vi "Get Digital Pattern - Multi FPGA.vi"(8 "error in (no error)":errorcluster, 11 "Item Ref in":T1 format="%.0x") -> (0 "error out":errorcluster, 2 "EPT Pattern":T2, 3 "Item Ref out":T1 format="%.0x")   [LabVIEW 2019, in "Engine Simulation Toolkit System Explorer.lvlib"]
uses:
  Engine Simulation Toolkit System Explorer.lvlib
  <vilib>/NI VeriStand/Custom Device API/Custom Device Item Ref.ctl
  Digital Pattern.ctl
  Digital Pattern Base.ctl
  Digital Pattern Remove Edge.ctl
  Digital Pattern Add Pulse.ctl
  Shared/Properties.vi
  <vilib>/NI VeriStand/Custom Device API/Get Item Property (Double).vi
  <vilib>/NI VeriStand/Custom Device API/Get Item Property (U16).vi
  <vilib>/NI VeriStand/Custom Device API/Get Item Property (String).vi
  <vilib>/NI VeriStand/Custom Device API/Get Item Property (Boolean).vi
  <vilib>/NI VeriStand/Custom Device API/Custom Device API.lvlib
  Shared/Engine Simulation Toolkit Shared.lvlib
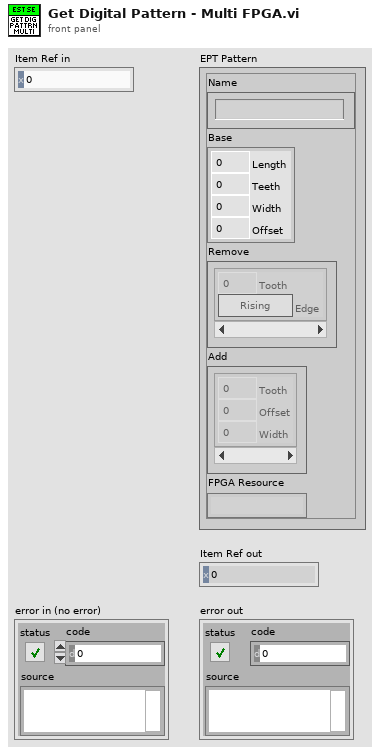
[diagram p1: front panel]
types:
  T1 = typedef "Custom Device API.lvlib/Custom Device Item Ref.ctl" = u64
  T2 = typedef "Engine Simulation Toolkit System Explorer.lvlib/Digital Pattern.ctl" = cluster{"Name":string, "Base":T3, "Remove":T4[], "Add":T5[], "FPGA Resource":string}
  T3 = typedef "Engine Simulation Toolkit System Explorer.lvlib/Digital Pattern Base.ctl" = cluster{"Length":dbl, "Teeth":u16, "Width":dbl, "Offset":dbl}
  T4 = typedef "Engine Simulation Toolkit System Explorer.lvlib/Digital Pattern Remove Edge.ctl" = cluster{"Tooth":u16, "Edge":bool}
  T5 = typedef "Engine Simulation Toolkit System Explorer.lvlib/Digital Pattern Add Pulse.ctl" = cluster{"Tooth":u16, "Offset":dbl, "Width":dbl}
  T6 = typedef "Custom Device API.lvlib/Custom Device Item Info.ctl" = cluster{"Name":string, "Is Channel":bool, "GUID":string, "Is Waveform":bool}
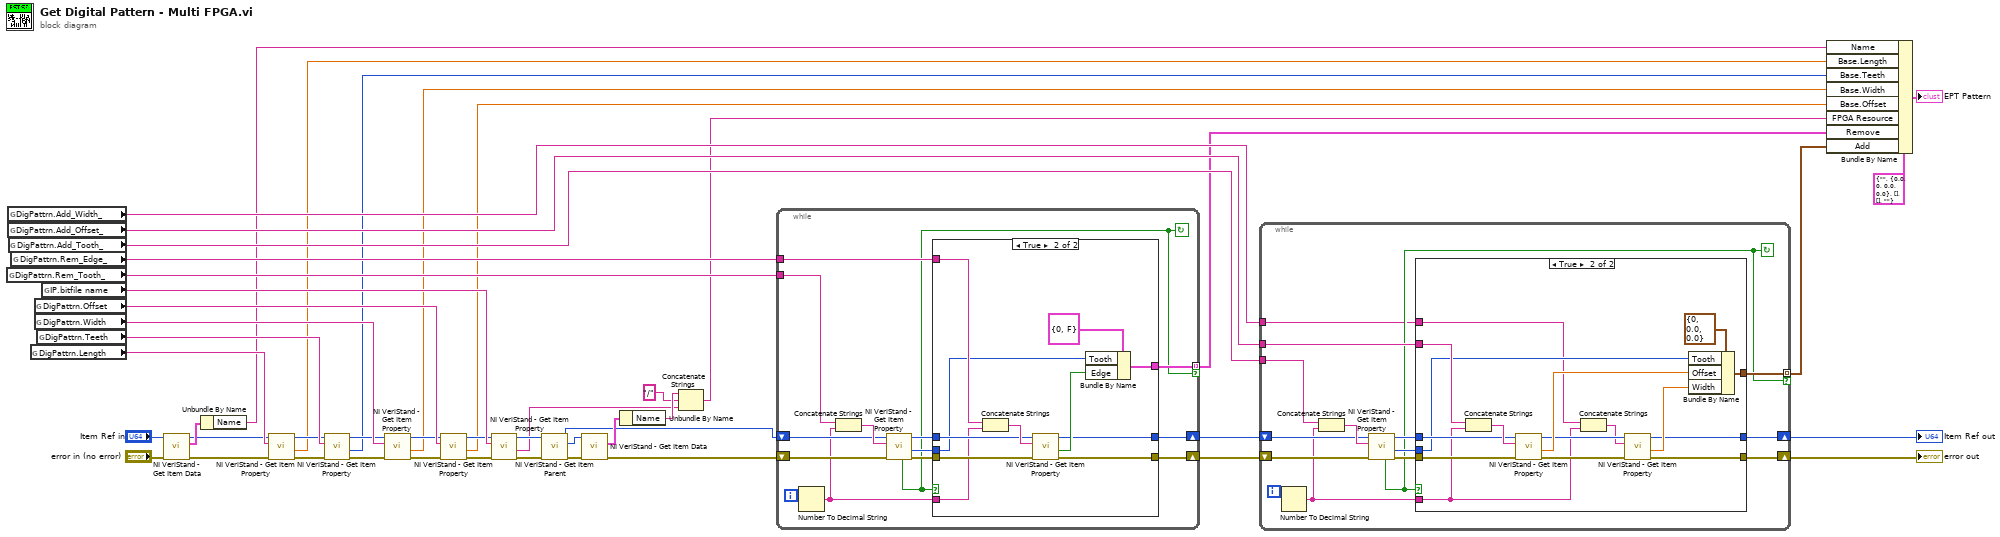
[diagram p0: block diagram]
diagram:
  n1 = global read "Properties.vi" "DigPattrn.Rem_Tooth_"() -> (w43:string)
  n2 = global read "Properties.vi" "DigPattrn.Add_Width_"() -> (w47:string)
  n3 = global read "Properties.vi" "DigPattrn.Add_Offset_"() -> (w46:string)
  n4 = global read "Properties.vi" "DigPattrn.Add_Tooth_"() -> (w45:string)
  n5 = global read "Properties.vi" "DigPattrn.Rem_Edge_"() -> (w44:string)
  n6 = global read "Properties.vi" "DigPattrn.Length"() -> (w38:string)
  n7 = global read "Properties.vi" "DigPattrn.Offset"() -> (w41:string)
  n8 = global read "Properties.vi" "DigPattrn.Width"() -> (w40:string)
  n9 = global read "Properties.vi" "DigPattrn.Teeth"() -> (w39:string)
  n10 = global read "Properties.vi" "IP.bitfile name"() -> (w42:string)
  n11 = call <vilib>:"NI VeriStand - Get Item Data.vi"("error in (no error)"="error in (no error)", "Item Ref in"="Item Ref in") -> ("error out"=w14:errorcluster, "Item Info"=w17:T6, "Item Ref out"=w15:T1)  [unwired: 6 in, 1 out]
  n12 = Unbundle By Name(w17) -> ("Name"=w36:string)
  n13 = call-poly <vilib>:"NI VeriStand - Get Item Property.vi"("error in (no error)"=w14, "Property Name"=w38, "Item Ref in"=w15) -> ("error out"=w22:errorcluster, "Value"=w20:dbl, "Item Ref out"=w21:T1)  [unwired: 5 in, 1 out]
  n14 = call-poly <vilib>:"NI VeriStand - Get Item Property.vi"("error in (no error)"=w22, "Property Name"=w39, "Item Ref in"=w21) -> ("error out"=w25:errorcluster, "Value"=w23:u16, "Item Ref out"=w24:T1)  [unwired: 5 in, 1 out]
  n15 = call-poly <vilib>:"NI VeriStand - Get Item Property.vi"("error in (no error)"=w25, "Property Name"=w40, "Item Ref in"=w24) -> ("error out"=w28:errorcluster, "Value"=w26:dbl, "Item Ref out"=w27:T1)  [unwired: 5 in, 1 out]
  n16 = call-poly <vilib>:"NI VeriStand - Get Item Property.vi"("error in (no error)"=w28, "Property Name"=w41, "Item Ref in"=w27) -> ("error out"=w35:errorcluster, "Value"=w29:dbl, "Item Ref out"=w34:T1)  [unwired: 5 in, 1 out]
  n17 = call-poly <vilib>:"NI VeriStand - Get Item Property.vi"("error in (no error)"=w35, "Property Name"=w42, "Item Ref in"=w34) -> ("error out"=w9:errorcluster, "Value"=w3:string, "Item Ref out"=w7:T1)  [unwired: 5 in, 1 out]
  n18 = call <vilib>:"NI VeriStand - Get Item Parent.vi"("error in (no error)"=w9, "Item Ref in"=w7) -> ("error out"=w11:errorcluster, "Parent Ref"=w6:T1, "Item Ref out"=w5:T1)  [unwired: 6 in, 1 out]
  n19 = call <vilib>:"NI VeriStand - Get Item Data.vi"("error in (no error)"=w11, "Item Ref in"=w6) -> ("error out"=w8:errorcluster, "Item Info"=w10:T6)  [unwired: 6 in, 2 out]
  n20 = Unbundle By Name(w10) -> ("Name"=w4:string)
  n21 = Concatenate Strings(w4, "/" ("string"), w3) -> (w1:string)
  n22 = while {
    shift-right: [w48] -> w32
    shift-left: w8 -> [w59]
    shift-right: [w49] -> w31
    shift-left: w5 -> [w60]
    tunnel: w44 -> [w54]
    tunnel: w43 -> [w52]
    tunnel: [w51] -> w30 mode=indexing if=w50
    i -> [w58]
    stop <- w50 continue-if-true
    n23 = Number To Decimal String(number=w58) -> (decimal integer string=w53:string)  [unwired: 1 in]
    n24 = Concatenate Strings(w52, w53) -> (w61:string)
    n25 = call-poly <vilib>:"NI VeriStand - Get Item Property.vi"("error in (no error)"=w59, "Property Name"=w61, "Item Ref in"=w60) -> ("error out"=w57:errorcluster, "Value"=w55:u16, "Item Ref out"=w56:T1, "Found?"=w50:bool)  [unwired: 5 in]
    n26 = case shown="True" w50 {
      tunnel: w57 -> [w62 w71]
      tunnel: w56 -> [w63 w72]
      tunnel: w55 -> [_ w68]
      tunnel: w54 -> [_ w70]
      tunnel: w53 -> [_ w69]
      tunnel: [w62 w66] -> w48
      tunnel: [w63 w65] -> w49
      tunnel: [_ w64] -> w51
      frame False {
      }
      frame True {
        n27 = Concatenate Strings(w70, w69) -> (w73:string)
        n28 = call-poly <vilib>:"NI VeriStand - Get Item Property.vi"("error in (no error)"=w71, "Property Name"=w73, "Item Ref in"=w72) -> ("error out"=w66:errorcluster, "Value"=w67:bool, "Item Ref out"=w65:T1)  [unwired: 5 in, 1 out]
        n29 = Bundle By Name(cluster=T4 {"Tooth"=0, "Edge"=FALSE} ("Remove Edge"), "Tooth"=w68, "Edge"=w67) -> (w64:T4)
      }
    }
  }
  n30 = while {
    shift-right: [w76] -> w18
    shift-left: w32 -> [w87]
    shift-right: [w77] -> w37
    shift-left: w31 -> [w88]
    tunnel: w46 -> [w82]
    tunnel: w45 -> [w80]
    tunnel: [w79] -> w33 mode=indexing if=w78
    tunnel: w47 -> [w75]
    i -> [w86]
    stop <- w78 continue-if-true
    n31 = Number To Decimal String(number=w86) -> (decimal integer string=w81:string)  [unwired: 1 in]
    n32 = Concatenate Strings(w80, w81) -> (w89:string)
    n33 = call-poly <vilib>:"NI VeriStand - Get Item Property.vi"("error in (no error)"=w87, "Property Name"=w89, "Item Ref in"=w88) -> ("error out"=w85:errorcluster, "Value"=w83:u16, "Item Ref out"=w84:T1, "Found?"=w78:bool)  [unwired: 5 in]
    n34 = case shown="True" w78 {
      tunnel: w85 -> [w90 w104]
      tunnel: w84 -> [w91 w105]
      tunnel: w83 -> [_ w102]
      tunnel: w82 -> [_ w103]
      tunnel: w81 -> [_ w93]
      tunnel: [w90 w97] -> w76
      tunnel: [w91 w95] -> w77
      tunnel: [_ w100] -> w79
      tunnel: w75 -> [_ w94]
      frame False {
      }
      frame True {
        n35 = Concatenate Strings(w103, w93) -> (w106:string)
        n36 = call-poly <vilib>:"NI VeriStand - Get Item Property.vi"("error in (no error)"=w104, "Property Name"=w106, "Item Ref in"=w105) -> ("error out"=w98:errorcluster, "Value"=w101:dbl, "Item Ref out"=w99:T1)  [unwired: 5 in, 1 out]
        n37 = Concatenate Strings(w94, w93) -> (w92:string)
        n38 = call-poly <vilib>:"NI VeriStand - Get Item Property.vi"("error in (no error)"=w98, "Property Name"=w92, "Item Ref in"=w99) -> ("error out"=w97:errorcluster, "Value"=w96:dbl, "Item Ref out"=w95:T1)  [unwired: 5 in, 1 out]
        n39 = Bundle By Name(cluster=T5 {"Tooth"=0, "Offset"=0.0, "Width"=0.0} ("Add Pulse"), "Tooth"=w102, "Offset"=w101, "Width"=w96) -> (w100:T5)
      }
    }
  }
  "Item Ref out" <- w37
  "error out" <- w18
  n40 = Bundle By Name(cluster=T2 {"Name"="", "Base"={"Length"=0.0, "Teeth"=0, "Width"=0.0, "Offset"=0.0}, "Remove"=[], "Add"=[], "FPGA Resource"=""} ("EPT Pattern"), "Name"=w36, "Base.Length"=w20, "Base.Teeth"=w23, "Base.Width"=w26, "Base.Offset"=w29, "FPGA Resource"=w1, "Remove"=w30, "Add"=w33) -> (→"EPT Pattern":T2)
